vi "Force Icon Editor to Unload.vi"() -> ()   [LabVIEW 2024]
panel:
  out "name found in memory":string
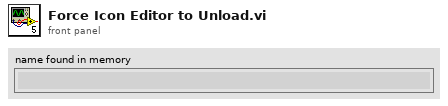
[diagram p1: front panel]
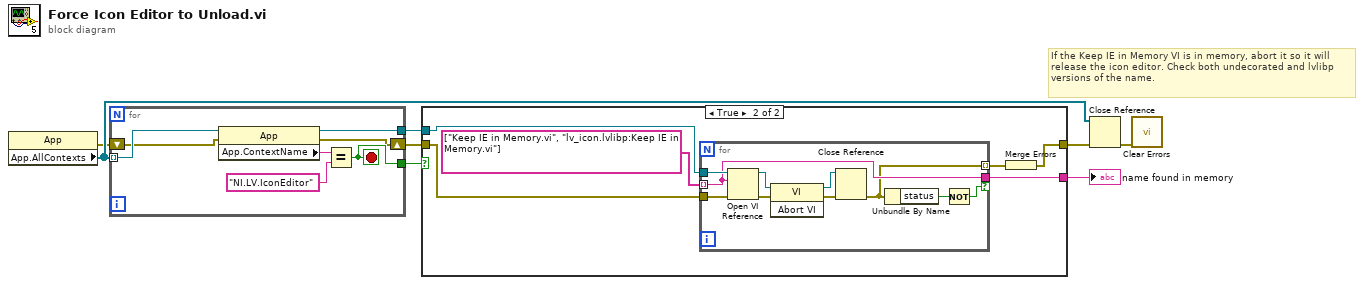
[diagram p0: block diagram]
diagram:
  # "If the Keep IE in Memory VI is in memory, abort it so it will release the icon editor. Check both undecorated and lvlibp versions of the name."
  n1 = property class="App"() -> (error out=w5:errorcluster, "App.AllContexts"=w8:refnum<vi>[])  [unwired: 2 in, 1 out]
  n2 = for {
    tunnel: w8 -> [w15] mode=indexing
    tunnel: [w14] -> w2
    tunnel: [w11] -> w4
    shift-right: [w9] -> w7
    shift-left: w5 -> [w10]
    stop <- w11 stop-if-true
    n3 = property class="App"(reference=w15, error in=w10) -> (reference out=w14:refnum<vi>, error out=w9:errorcluster, "App.ContextName"=w13:string)
    n4 = Equal?(x=w13, y="NI.LV.IconEditor" ("machine name (\"\":  open local reference)")) -> (x = y?=w11:bool)
  }
  n5 = case shown="True" w4 {
    tunnel: w2 -> [_ w22]
    tunnel: [w16 w18] -> w6
    tunnel: w7 -> [w16 w20]
    tunnel: [_ w17] -> w1
    frame False {
    }
    frame True {
      n6 = for {
        tunnel: w22 -> [w31]
        tunnel: string[] ["Keep IE in Memory.vi", "lv_icon.lvlibp:Keep IE in Memory.vi"] -> [w26] mode=indexing
        tunnel: w20 -> [w30]
        tunnel: [w25] -> w21 mode=indexing
        tunnel: [w26] -> w17 if=w23
        n7 = Open VI Reference(application reference (local)=w31, vi path=w26, error in (no error)=w30) -> (vi reference=w32:refnum<vi>, error out=w27:errorcluster)  [unwired: 3 out]
        n8 = invoke class="VI" method="Abort VI"(reference=w32, error in=w27) -> (reference out=w29:refnum<vi>, error out=w28:errorcluster)  [unwired: 1 in, 1 out]
        n9 = Close Reference(reference=w29, error in (no error)=w28) -> (error out=w25:errorcluster)
        n10 = Unbundle By Name(w25) -> ("status"=w24:bool)
        n11 = Not(x=w24) -> (.not. x?=w23:bool)
      }
      n12 = Merge Errors(w21) -> (w18:errorcluster)
    }
  }
  "name found in memory" <- w1
  n13 = Close Reference(reference=w8, error in (no error)=w6) -> (error out=w3:errorcluster)
  n14 = call <vilib>:"Clear Errors.vi"("error in (no error)"=w3) -> ()  [unwired: 5 in, 2 out]
